vi "Read TDMS_CANFD.vi"() -> ()   [LabVIEW 2020]
uses:
  <vilib>/xnet/xnet.llb/XNET Frame CAN.ctl
  <vilib>/xnet/xnet.llb/XNET Frame Type CAN.ctl
  Program Files (x86)/National Instruments/LabVIEW 2020/examples/nixnet/NI-XNET Frame Conversion and Logfile.llb/NI-XNET Frame&Log - Convert Frames (Raw to CAN).vi
panel:
  out "data":u8[](array[numeric])
  out "size(s)":i32
  out "CAN frames":T1[](array[typedef])=[{"timestamp"=timestamp(3700018536.6760993 s since 1904-01-01), "payload"=[1, 2, 3, 4, 5, 6, 7, 8, 0, 0, 0, 0], "identifier"=8, "type"=16, "extended?"=FALSE, "echo?"=FALSE}, {"timestamp"=timestamp(3700018576.8273134 s since 1904-01-01), "payload"=[1, 2, 3, 4, 5, 6, 7, 8, 0, 0, 0, 0, 0, 0, 0, 0, 0, 0, 0, 0, 0, 0, 0, 0, 0, 0, 0, 0, 0, 0, 0, 0, 0, 0, 0, 0, 0, 0, 0, 0, 0, 0, 0, 0, 0, 0, 0, 0, 0, 0, 0, 0, 0, 0, 0, 0, 0, 0, 0, 0, 0, 0, 0, 0], "identifier"=8, "type"=16, "extended?"=FALSE, "echo?"=FALSE}, {"timestamp"=timestamp(3700018596.821688 s since 1904-01-01), "payload"=[1, 2, 3, 4], "identifier"=8, "type"=16, "extended?"=FALSE, "echo?"=FALSE}] {"payload" format="%x"; "timestamp" format="%<%.7X\n%x>T"; "type" items=["CAN Data"=0, "CAN Remote"=1, "CAN Bus Error"=2, "CAN 2.0 Data"=8, "CAN FD Data"=16, "CAN FD+BRS Data"=24, "J1939 Data"=192, "Delay"=224, "Log Trigger"=225, "Start Trigger"=226]; "identifier" format="%x"}
  in  "Group Name":string="My Group"
  in  "Channel Name":string="My Channel"
  in  "TDMS Logfile Path":path=path "C:/Users/kvemishe/Documents/Rivian/Replay/CAN/XnetBmLogFD.tdms"
  out "Reading TDMS File":bool=TRUE
  in  "Number of Frames to Read (-1:all)":i64=-1
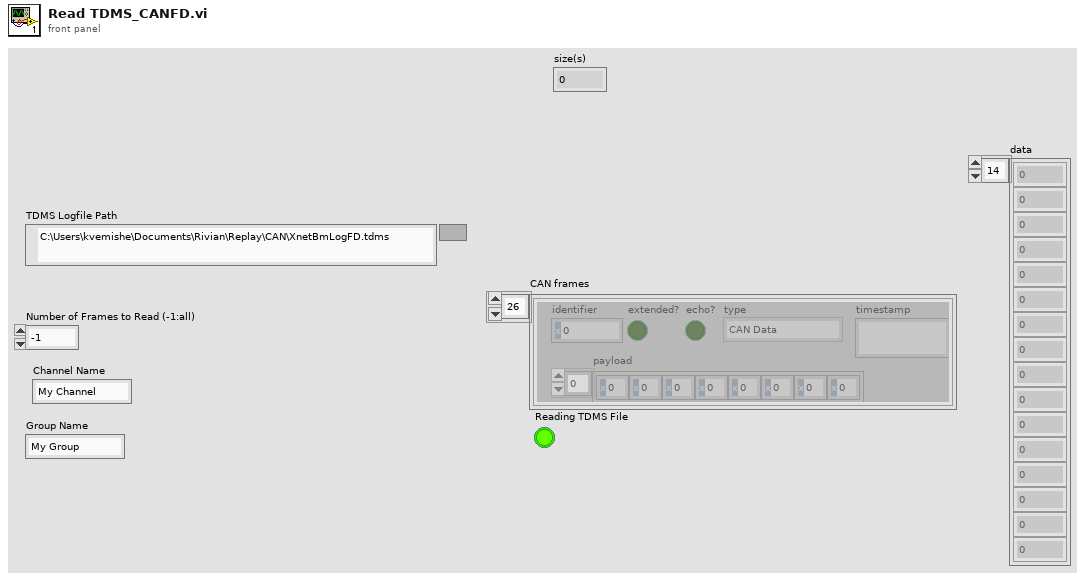
[diagram p1: front panel]
types:
  T1 = typedef "XNET Frame CAN.ctl" = cluster{"timestamp":timestamp, "payload":u8[], "identifier":u32, "type":T2, "extended?":bool, "echo?":bool}
  T2 = typedef "XNET Frame Type CAN.ctl" = u8
  T3 = enum16{"open", "open or create", "create or replace", "create", "open (read-only)"}
  T4 = typedef "NI-XNET Frame&Log - Converter.ctl" = cluster{"endian swap?":bool, "partial":u8[], "index":i32}
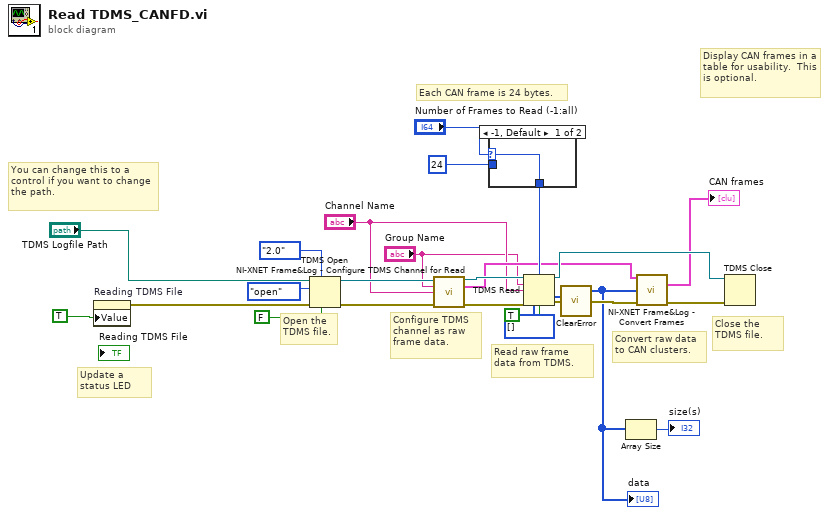
[diagram p0: block diagram]
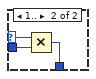
[diagram p2: hidden frame]
diagram:
  # "Each CAN frame is 24 bytes."
  # "Convert raw data\nto CAN clusters."
  # "Configure TDMS\nchannel as raw \nframe data."
  # "Close the TDMS file."
  # "Read raw frame\ndata from TDMS."
  # "Open the \nTDMS file."
  # "You can change this to a control if you want to change the path."
  # "Update a status LED"
  # "Display CAN frames in a table for usability.  This is optional."
  n1 = property on="Reading TDMS File" class="Bool (strict)"("Value"=TRUE ("Reading NCL File")) -> (error out=w14:errorcluster)  [unwired: 2 in, 1 out]
  n2 = TDMS Open(6:FALSE ("disable buffering (T)"), 7:enum16{"1.0", "2.0"}."2.0" ("file format version (2.0)"), 8:w14, 10:T3."open" ("operation (0:open)"), 11:"TDMS Logfile Path") -> (0:w23:errorcluster, 3:w22:refnum<k34>)  [unwired: 2 in]
  n3 = call "NI-XNET Frame&Log - Configure TDMS Channel for Read.vi"("tdms file in"=w22, "group name (Untitled)"="Group Name", "channel name"="Channel Name", "error in (no error)"=w23) -> ("tdms file out"=w21:refnum<k34>, "converter"=w10:T4, "error out"=w20:errorcluster)  [unwired: 7 in, 2 out]
  n4 = case shown="-1, Default" "Number of Frames to Read (-1:all)" {
    selector: "Number of Frames to Read (-1:all)" -> [w26 w27]
    tunnel: i64 24 ("y") -> [_ w29]
    tunnel: [w26 w28] -> w12
    frame -1, Default {
    }
    frame 1.. {
      n5 = Multiply(x=w27, y=w29) -> (x*y=w28:i64)
    }
  }
  n6 = TDMS Read(0:w21, 2:w12, 5:"Group Name", 7:"Channel Name", 11:w20, 12:u8[] [] ("raw frames"), 13:TRUE ("return channels in file order? (F)")) -> (4:w17:refnum<k34>, 10:w2:u8[], 15:w9:errorcluster)  [unwired: 1 in, 3 out]
  "data" <- w2
  n7 = call <vilib>:"ClearError.vi"("error in (no error)"=w9) -> ("error out"=w19:errorcluster)
  n8 = Array Size(array=w2) -> (size(s)=→"size(s)":i32)
  n9 = call-poly "NI-XNET Frame&Log - Convert Frames.vi"("converter in"=w10, "raw frames"=w2, "error in"=w19) -> ("CAN frames"=→"CAN frames":T1[], "error out"=w18:errorcluster)  [unwired: 11 out]
  n10 = TDMS Close(8:w18, 11:w17) -> ()  [unwired: 2 out]
